vi "1.vi"() -> ()   [LabVIEW 2019]
panel:
  out "Output":dbl
  in  "B":dbl
  in  "A":dbl
  in  "Button":bool
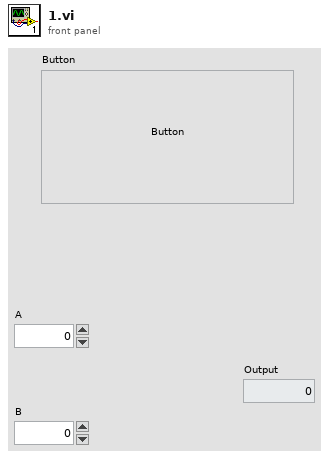
[diagram p1: front panel]
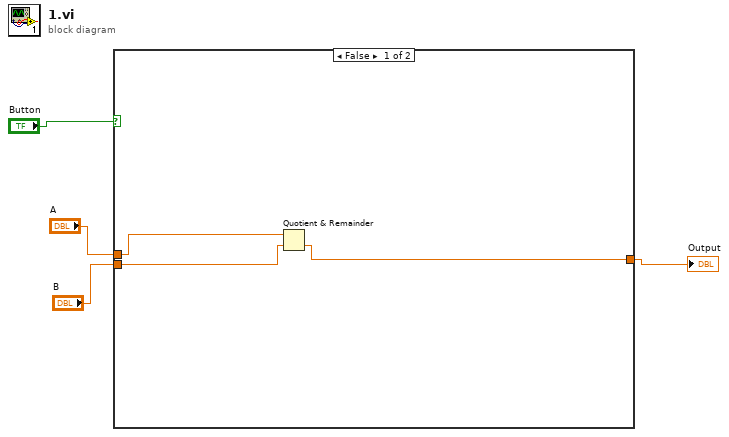
[diagram p0: block diagram]
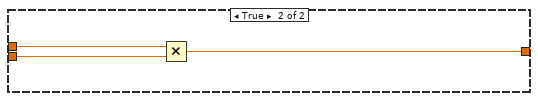
[diagram p2: hidden frame]
diagram:
  n1 = case shown="False" "Button" {
    tunnel: "A" -> [w7 w10]
    tunnel: "B" -> [w6 w9]
    tunnel: [w5 w8] -> w1
    frame False {
      n2 = Quotient & Remainder(x=w7, y=w6) -> (floor(x/y)=w5:dbl)  [unwired: 1 out]
    }
    frame True {
      n3 = Multiply(x=w10, y=w9) -> (x*y=w8:dbl)
    }
  }
  "Output" <- w1
